vi "ActionVIOnCompile.vi"(8 "error in (no error)":errorcluster, 11 "Device Item Ref in":T4 format="%.0x") -> (0 "error out":errorcluster)   [LabVIEW 2015, in "SLSC EDS System Explorer.lvlib"]
uses:
  SLSC EDS System Explorer.lvlib
  <vilib>/NI Veristand/Custom Device API/Custom Device Item Ref.ctl
  SLSC CD API/SLSC CD Engine/SLSC Dynamic Channel.ctl
  SLSC CD API/SLSC CD Engine/SLSC Datatype.ctl
  Shared/Compiled.Settings
  Shared/SLSC Static Settings.ctl
  Shared/Constants.vi
  <vilib>/NI Veristand/Custom Device API/Get Item Property (Boolean).vi
  <vilib>/NI Veristand/Custom Device Tools/Custom Device Utility Library/NI VeriStand - Search for Item by Name.vi
  <vilib>/NI Veristand/Custom Device API/Get Item Property (I32).vi
  <vilib>/NI Veristand/Custom Device API/Get Item Property (U32).vi
  <vilib>/NI Veristand/Custom Device API/Get Item Property (String).vi
  <vilib>/NI Veristand/Custom Device Tools/Custom Device Utility Library/NI VeriStand - Search for All Items by Name.vi
  <vilib>/NI Veristand/Custom Device API/Set Item Property (Variant).vi
  <vilib>/NI VeriStand/Custom Device Tools/Custom Device Utility Library/Custom Device Utility Library.lvlib
  <vilib>/NI VeriStand/Custom Device API/Custom Device API.lvlib
  <vilib>/NI/NIVS Inline Async API/_Data Access System Explorer/Data Access System Explorer.lvlib
  Shared/SLSC EDS Shared.lvlib
  SLSC CD API/SLSC CD Shared/SLSC CD Shared.lvlib
  SLSC CD API/SLSC CD System Explorer/SLSC CD System Explorer.lvlib
panel:
  out "appended array":T1(array[cluster])
  out "SLSC Commands":T2[](array[typedef])
  out "SLSC Set/Write Properties":T2[](array[typedef])
  out "SLSC Get/Read Properties":T2[](array[typedef])
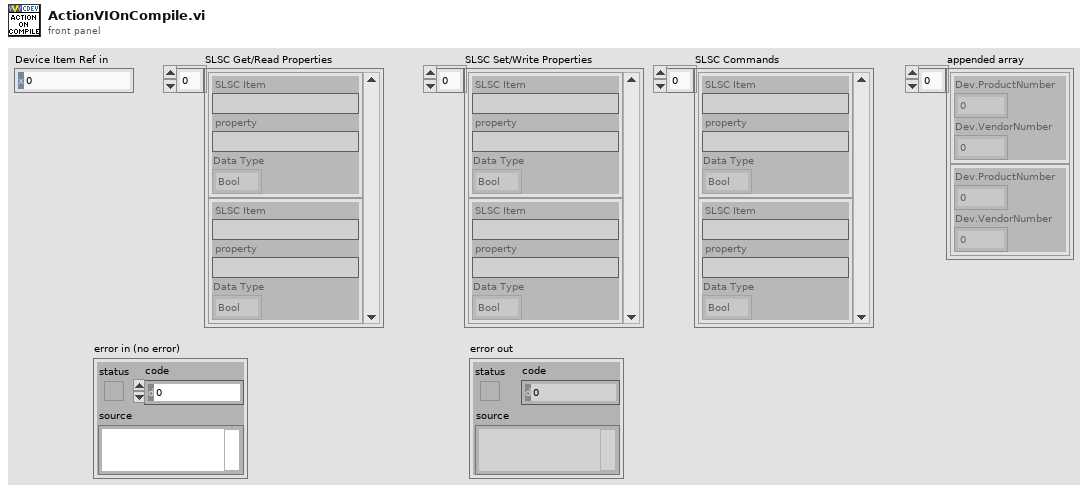
[diagram p1: front panel]
types:
  T1 = cluster{"Dev.ProductNumber":u32, "Dev.VendorNumber":u32}[]
  T2 = typedef "SLSC CD Shared.lvlib/SLSC Dynamic Channel.ctl" = cluster{"SLSC Item":string, "property":string, "Data Type":T3}
  T3 = typedef "SLSC CD Shared.lvlib/SLSC Datatype.ctl" = enum16{"Bool", "Double", "I32", "I64", "String", "U32", "U64"}
  T4 = typedef "Custom Device API.lvlib/Custom Device Item Ref.ctl" = u64
  T5 = cluster{"Dev.ProductNumber":u32, "Dev.VendorNumber":u32}
  T6 = enum16{"Output/Write", "Input/Read", "Input/ReadWrite"}
  T7 = typedef "SLSC EDS Shared.lvlib/Compiled.Settings" = cluster{"Name":string, "SLSC Name or IP Address":string, "Slot #":i32, "Configuration Data":T8, "SLSC Get/Read Properties":T2[], "SLSC Set/Write Properties":T2[], "SLSC Dynamic Commands":T2[], "Support Modules":cluster{"Dev.ProductNumber":u32, "Dev.VendorNumber":u32}[]}
  T8 = typedef "SLSC EDS Shared.lvlib/SLSC Static Settings.ctl" = cluster{"Properties":cluster{"Boolean Properties":cluster{"property":refnum<k21>, "Value":bool, "SLSC Item":refnum<k21>, "reset value":bool}[], "Double Properties":cluster{"property":refnum<k21>, "Double Write":dbl, "SLSC Item":refnum<k21>, "Double Reset Value":dbl}[], "I32 Properties":cluster{"property":refnum<k21>, "Int32 Write":i32, "SLSC Item":refnum<k21>, "Int32 Reset Value":i32}[], "I64 Properties":cluster{"property":refnum<k21>, "Int64 Write":i64, "SLSC Item":refnum<k21>, "Int64 Reset Value":i64}[], "String Properties":cluster{"property":refnum<k21>, "String Write":string, "SLSC Item":refnum<k21>, "String Reset Value":string}[], "U32 Properties":cluster{"property":refnum<k21>, "UInt32 Write":u32, "SLSC Item":refnum<k21>, "UInt32 Reset Value":u32}[], "U64 Properties":cluster{"property":refnum<k21>, "UInt64 Write":u64, "SLSC Item":refnum<k21>, "UInt64 Reset Value":u64}[]}, "Commands":T2[], "Reset Commands":T2[], "Apply Values on Deployment":bool, "Apply Reset on Undeployment":bool}
  T9 = cluster{"Name":string, "Type":enum16{"Output/Write", "Input/Read", "Input/ReadWrite"}, "VS Refs":T4[]}
  T10 = typedef "Custom Device API.lvlib/Custom Device Item Info.ctl" = cluster{"Name":string, "Is Channel":bool, "GUID":string, "Is Waveform":bool}
  T11 = typedef "EDSjsonStructure.ctl" = cluster{"vendorNum":u32, "vendorName":string, "vendorPrefix":string, "productNum":u32, "productName":string, "capsVersion":string, "capsSpecVersion":u32, "capsSpecOldestCompatibleVersion":u32, "enums":T12[], "properties":T13[], "commands":T14[], "scales":T15[], "physicalChannels":T16[], "registerMap":cluster{"registers":T17[]}}
  T12 = typedef "enum.ctl" = cluster{"name":string, "description-en":string, "values":cluster{"name":string, "description-en":string, "value":i32}[]}
  T13 = typedef "property.ctl" = cluster{"name":string, "description-en":string, "documentation-en":string, "dataType":string, "bitfield":string, "access":string, "scale":string, "value":variant, "min":variant, "max":variant, "default value":variant}
  T14 = typedef "command.ctl" = cluster{"name":string, "description-en":string, "documentation-en":string, "startBitfield":string, "waitTimeInMs":i32, "doneBitfield":string, "doneInterrupt":string, "doneTimeoutInMs":i32, "value":variant}
  T15 = typedef "scale.ctl" = cluster{"name":string, "description-en":string, "m":dbl, "b":dbl, "forwardCoeffs":dbl[], "reverseCoeffs":dbl[], "coercion":string, "table":cluster{"scaled":dbl, "unscaled":dbl}[]}
  T16 = typedef "physicalChannel.ctl" = cluster{"name":string, "description-en":string, "commands":T14[], "properties":T13[]}
  T17 = typedef "register.ctl" = cluster{"name":string, "description-en":string, "access":string, "address":u32, "size":u32, "bitfields":cluster{"name":string, "description-en":string, "offset":u32, "size":u32, "signed":bool, "strobe":bool}[]}
  T18 = cluster{"Name":string, "Type":enum16{"Output/Write", "Input/Read", "Input/ReadWrite"}, "VS Refs":T4[]}[]
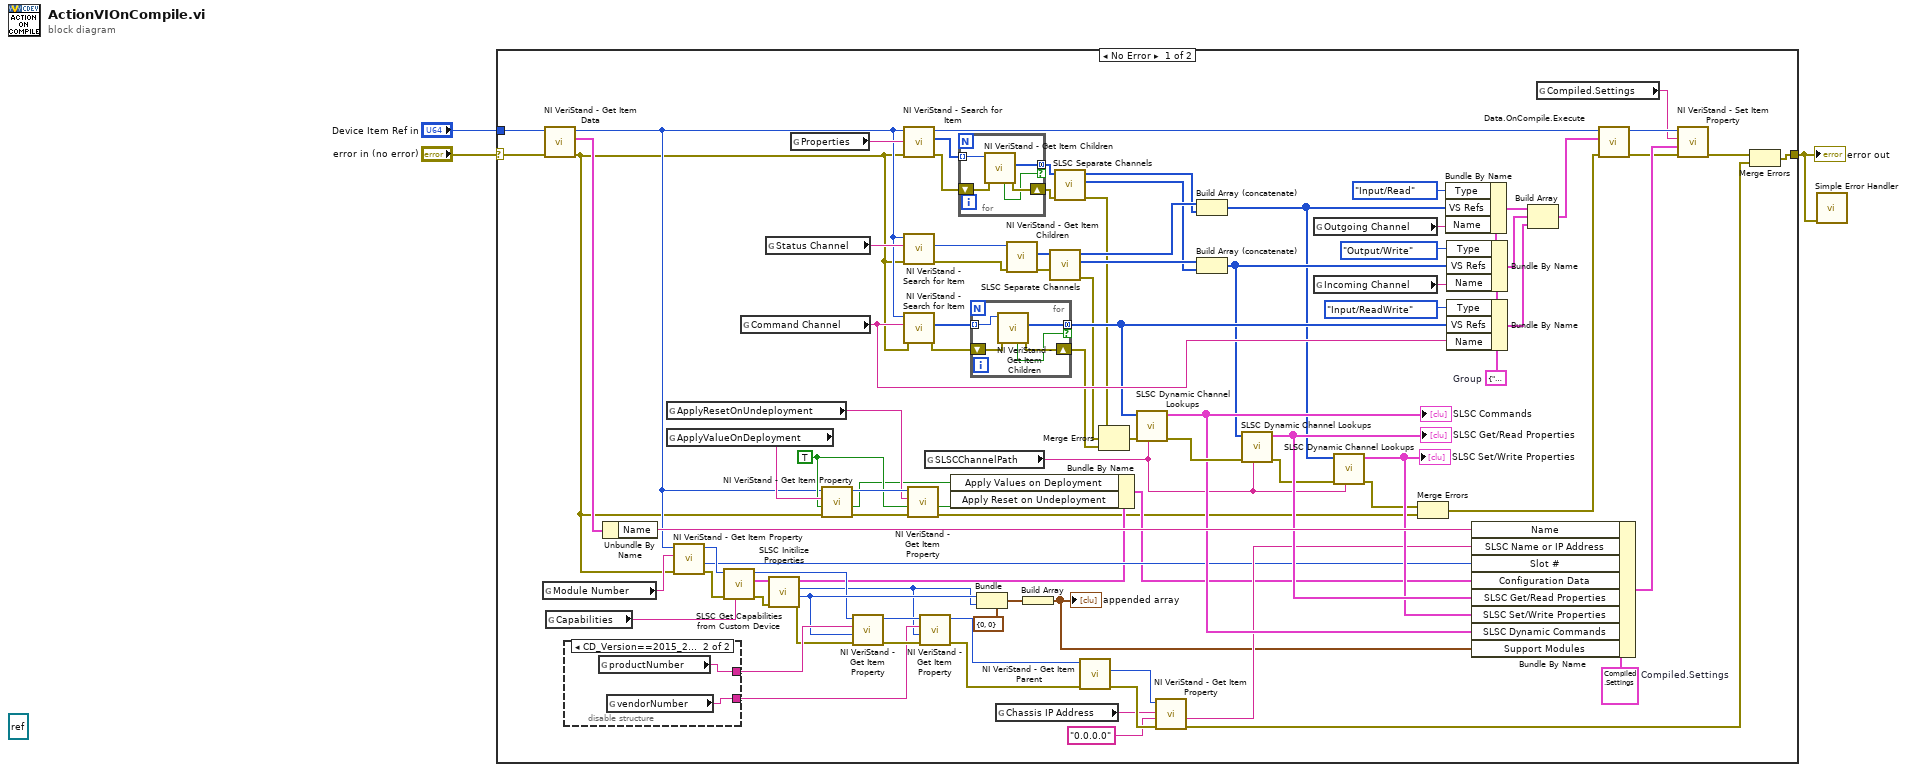
[diagram p0: block diagram]
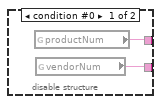
[diagram p2: hidden frame]
diagram:
  (unwired) refnum<k7> refnum ("SHDocVw.IWebBrowser2")
  n1 = case shown="No Error" "error in (no error)" {
    selector: "error in (no error)" -> [w78 w110]
    tunnel: [w76 w110] -> w1
    tunnel: "Device Item Ref in" -> [w79 _]
    frame No Error {
      w14 = TRUE ("Default Value")
      w71 = T7 {"Name"="", "SLSC Name or IP Address"="", "Slot #"=0, "Configuration Data"={"Properties"={"Boolean Properties"=[], "Double Properties"=[], "I32 Properties"=[], "I64 Properties"=[], "String Properties"=[], "U32 Properties"=[], "U64 Properties"=[]}, "Commands"=[], "Reset Commands"=[], "Apply Values on Deployment"=TRUE, "Apply Reset on Undeployment"=TRUE}, "SLSC Get/Read Properties"=[], "SLSC Set/Write Properties"=[], "SLSC Dynamic Commands"=[], "Support Modules"=[]}  # Compiled.Settings
      w63 = T9 {"Name"="", "Type"=enum."Output/Write", "VS Refs"=[]}  # Group
      n2 = global read "Constants.vi" "Module Number"() -> (w81:string)
      n3 = call <vilib>:"NI VeriStand - Get Item Data.vi"("error in (no error)"=w78, "Item Ref in"=w79) -> ("error out"=w8:errorcluster, "Item Info"=w92:T10, "Item Ref out"=w13:T4)  [unwired: 6 in, 1 out]
      n4 = global read "Constants.vi" "Capabilities"() -> (w4:string)
      n5 = disable-structure shown="CD_Version==2015_2016" {
        disable-tunnel: [w97 w99] -> w33
        disable-tunnel: [w96 w98] -> w32
        frame condition #0 {
          n6 = global read "Constants.vi" "productNum"() -> (w97:string)
          n7 = global read "Constants.vi" "vendorNum"() -> (w96:string)
        }
        frame condition #1 (active) {
          n8 = global read "Constants.vi" "productNumber"() -> (w99:string)
          n9 = global read "Constants.vi" "vendorNumber"() -> (w98:string)
        }
      }
      n10 = Unbundle By Name(w92) -> ("Name"=w91:string)
      n11 = global read "Constants.vi" "ApplyResetOnUndeployment"() -> (w16:string)
      n12 = global read "Constants.vi" "ApplyValueOnDeployment"() -> (w18:string)
      n13 = call-poly <vilib>:"NI VeriStand - Get Item Property.vi"("error in (no error)"=w8, "Property Name"=w81, "Item Ref in"=w13) -> ("error out"=w21:errorcluster, "Value"=w22:i32, "Item Ref out"=w25:T4)  [unwired: 5 in, 1 out]
      n14 = call "SLSC Get Capabilities from Custom Device.vi"("Property Name"=w4, "error in (no error)"=w21, "Device Item Ref in"=w25) -> ("error out"=w20:errorcluster, "data"=w24:T11, "Item Ref out"=w23:T4)  [unwired: 6 in]
      n15 = global read "Constants.vi" "Command Channel"() -> (w64:string)
      n16 = global read "Constants.vi" "Status Channel"() -> (w68:string)
      n17 = call "SLSC Initilize Properties.vi"("error in (no error)"=w20, "Capabilities"=w24) -> ("error out"=w26:errorcluster, "productNum"=w28:u32, "vendorNum"=w19:u32, "Configuration Data"=w12:T8)  [unwired: 5 in, 1 out]
      n18 = global read "Constants.vi" "Properties"() -> (w73:string)
      n19 = call-poly <vilib>:"NI VeriStand - Get Item Property.vi"("error in (no error)"=w8, "Default Value"=w14, "Property Name"=w18, "Item Ref in"=w13) -> ("error out"=w15:errorcluster, "Value"=w10:bool, "Item Ref out"=w17:T4)  [unwired: 4 in, 1 out]
      n20 = call-poly <vilib>:"NI VeriStand - Get Item Property.vi"("error in (no error)"=w26, "Default Value"=w28, "Property Name"=w33, "Item Ref in"=w23) -> ("error out"=w35:errorcluster, "Item Ref out"=w37:T4)  [unwired: 4 in, 2 out]
      n21 = call-poly <vilib>:"NI VeriStand - Search for Item.vi"("error in"=w8, "Item Name"=w73, "Section Ref in"=w13) -> ("error out"=w43:errorcluster, "Item Refs"=w95:T4[], "Section Ref out"=w51:T4)  [unwired: 5 in, 1 out]
      n22 = call-poly <vilib>:"NI VeriStand - Search for Item.vi"("error in"=w8, "Item Name"=w68, "Section Ref in"=w13) -> ("error out"=w70:errorcluster, "Item Ref"=w69:T4)  [unwired: 5 in, 2 out]
      n23 = call-poly <vilib>:"NI VeriStand - Search for Item.vi"("error in"=w8, "Item Name"=w64, "Section Ref in"=w13) -> ("error out"=w66:errorcluster, "Item Refs"=w67:T4[])  [unwired: 5 in, 2 out]
      n24 = call-poly <vilib>:"NI VeriStand - Get Item Property.vi"("error in (no error)"=w15, "Default Value"=w14, "Property Name"=w16, "Item Ref in"=w17) -> ("error out"=w6:errorcluster, "Value"=w9:bool)  [unwired: 4 in, 2 out]
      n25 = call-poly <vilib>:"NI VeriStand - Get Item Property.vi"("error in (no error)"=w35, "Default Value"=w19, "Property Name"=w32, "Item Ref in"=w37) -> ("error out"=w34:errorcluster, "Item Ref out"=w36:T4)  [unwired: 4 in, 2 out]
      n26 = global read "Constants.vi" "SLSCChannelPath"() -> (w5:string)
      n27 = Bundle By Name(cluster=w12, "Apply Values on Deployment"=w10, "Apply Reset on Undeployment"=w9) -> (w11:T8)
      n28 = for {
        tunnel: w95 -> [w104] mode=indexing
        tunnel: [w102] -> w50 mode=concatenating if=w100
        shift-right: [w101] -> w45
        shift-left: w43 -> [w103]
        n29 = call <vilib>:"NI VeriStand - Get Item Children.vi"("error in (no error)"=w103, "Item Ref in"=w104) -> ("error out"=w101:errorcluster, "Child Refs"=w102:T4[], "Found"=w100:bool)  [unwired: 6 in, 1 out]
      }
      n30 = for {
        tunnel: w67 -> [w109] mode=indexing
        tunnel: [w106] -> w58 mode=concatenating if=w105
        shift-right: [w107] -> w62
        shift-left: w66 -> [w108]
        n31 = call <vilib>:"NI VeriStand - Get Item Children.vi"("error in (no error)"=w108, "Item Ref in"=w109) -> ("error out"=w107:errorcluster, "Child Refs"=w106:T4[], "Found"=w105:bool)  [unwired: 6 in, 1 out]
      }
      n32 = Bundle(cluster=T5 {"Dev.ProductNumber"=0, "Dev.VendorNumber"=0} ("Product Identification"), "Dev.ProductNumber"=w28, "Dev.VendorNumber"=w19) -> (w30:T5)
      n33 = global read "Constants.vi" "Chassis IP Address"() -> (w80:string)
      n34 = call <vilib>:"NI VeriStand - Get Item Children.vi"("error in (no error)"=w70, "Item Ref in"=w69) -> ("error out"=w44:errorcluster, "Child Refs"=w54:T4[])  [unwired: 6 in, 2 out]
      n35 = Build Array(w30) -> (w29:T1)
      "appended array" <- w29
      n36 = call "SLSC Separate Channels.vi"("error in (no error)"=w44, "Item Refs In"=w54) -> ("error out"=w41:errorcluster, "Output Channels"=w52:T4[], "Input Channels"=w53:T4[])  [unwired: 6 in, 1 out]
      n37 = call "SLSC Separate Channels.vi"("error in (no error)"=w45, "Item Refs In"=w50) -> ("error out"=w40:errorcluster, "Output Channels"=w48:T4[], "Input Channels"=w49:T4[])  [unwired: 6 in, 1 out]
      n38 = call <vilib>:"NI VeriStand - Get Item Parent.vi"("error in (no error)"=w34, "Item Ref in"=w36) -> ("error out"=w83:errorcluster, "Parent Ref"=w82:T4)  [unwired: 6 in, 2 out]
      n39 = Merge Errors(w40, w41, w62) -> (w60:errorcluster)
      n40 = call "SLSC Dynamic Channel Lookups.vi"("SLSCChannelPath"=w5, "error in (no error)"=w60, "Child Refs"=w58) -> ("error out"=w59:errorcluster, "SLSC Dynamic Inputs"=w57:T2[])  [unwired: 7 in]
      "SLSC Commands" <- w57
      n41 = call-poly <vilib>:"NI VeriStand - Get Item Property.vi"("error in (no error)"=w83, "Default Value"="0.0.0.0", "Property Name"=w80, "Item Ref in"=w82) -> ("error out"=w27:errorcluster, "Value"=w56:string)  [unwired: 4 in, 2 out]
      n42 = Build Array (concatenate)(w53, w49) -> (w38:T4[])
      n43 = Build Array (concatenate)(w52, w48) -> (w39:T4[])
      n44 = call "SLSC Dynamic Channel Lookups.vi"("SLSCChannelPath"=w5, "error in (no error)"=w59, "Child Refs"=w39) -> ("error out"=w74:errorcluster, "SLSC Dynamic Inputs"=w75:T2[])  [unwired: 7 in]
      "SLSC Get/Read Properties" <- w75
      n45 = global read "Constants.vi" "Outgoing Channel"() -> (w47:string)
      n46 = global read "Constants.vi" "Incoming Channel"() -> (w46:string)
      n47 = call "SLSC Dynamic Channel Lookups.vi"("SLSCChannelPath"=w5, "error in (no error)"=w74, "Child Refs"=w38) -> ("error out"=w42:errorcluster, "SLSC Dynamic Inputs"=w72:T2[])  [unwired: 7 in]
      "SLSC Set/Write Properties" <- w72
      n48 = Merge Errors(w42, w6) -> (w7:errorcluster)
      n49 = Bundle By Name(cluster=w63, "Type"=T6."Input/Read", "VS Refs"=w38, "Name"=w47) -> (w90:T9)
      n50 = Bundle By Name(cluster=w63, "Type"=T6."Output/Write", "VS Refs"=w39, "Name"=w46) -> (w86:T9)
      n51 = Bundle By Name(cluster=w63, "Type"=T6."Input/ReadWrite", "VS Refs"=w58, "Name"=w64) -> (w61:T9)
      n52 = Bundle By Name(cluster=w71, "Name"=w91, "SLSC Name or IP Address"=w56, "Slot #"=w22, "Configuration Data"=w11, "SLSC Get/Read Properties"=w75, "SLSC Set/Write Properties"=w72, "SLSC Dynamic Commands"=w57, "Support Modules"=w29) -> (w94:T7)
      n53 = Build Array(w90, w86, w61) -> (w88:T18)
      n54 = global read "Constants.vi" "Compiled.Settings"() -> (w77:string)
      n55 = call <vilib>:"Data.OnCompile.Execute.vi"("error in"=w7, "VS Ref Groups"=w88, "Custom Device Ref"=w51) -> ("error out"=w85:errorcluster, "Custom Device Ref"=w84:T4)  [unwired: 7 in]
      n56 = call-poly <vilib>:"NI VeriStand - Set Item Property.vi"("error in (no error)"=w85, "Value"=w94, "Property Name"=w77, "Item Ref in"=w84) -> ("error out"=w93:errorcluster)  [unwired: 5 in, 2 out]
      n57 = Merge Errors(w93, w27) -> (w76:errorcluster)
    }
    frame Error {
    }
  }
  "error out" <- w1
  n58 = call <vilib>:"Simple Error Handler.vi"("error in (no error)"=w1) -> ()  [unwired: 4 in, 5 out]
